vi "Initialize Session.vi"(8 "error in (no error)":errorcluster, 9 "Initialize_Info":T1, 10 "session reservation":refnum<class "Session Reservation.lvclass">, 11 "NI-DMM in":refnum<class "niDMM.lvclass">) -> (0 "error out":errorcluster, 3 "NI-DMM out":refnum<class "niDMM.lvclass">)   [LabVIEW 2021, in "niDMM.lvclass"]
uses:
  niDMM.lvclass
  TypeDefs/Initialize_Info.ctl
  <vilib>/Plug-In SDKs/Clients/Session Management V1/Session Reservation/Initialize and Close Session Behavior.ctl
  <vilib>/Plug-In SDKs/Clients/Session Management V1/Session Reservation/Session Reservation.lvclass
  niDMM.lvclass/niDMM.ctl
  <vilib>/Plug-In SDKs/Sessions/niDMM/Initialize Sessions - 1Sess.vi
  <vilib>/Plug-In SDKs/Sessions/niDMM/NI Session Management niDMM.lvlib
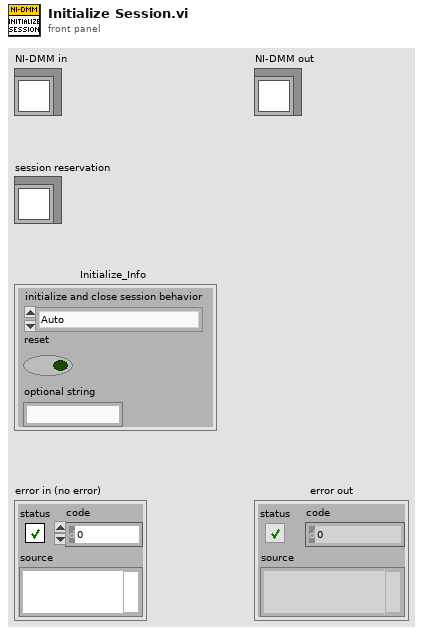
[diagram p1: front panel]
types:
  T1 = typedef "niDMM.lvclass/Initialize_Info.ctl" = cluster{"initialize and close session behavior":T2, "reset":bool, "optional string":string}
  T2 = typedef "NI Session Management V1 Client.lvlib/Session Reservation.lvclass/Initialize and Close Session Behavior.ctl" = enum16{"Auto", "Initialize and Close", "Attach and Detach", "Initialize and Detach", "Attach and Close"}
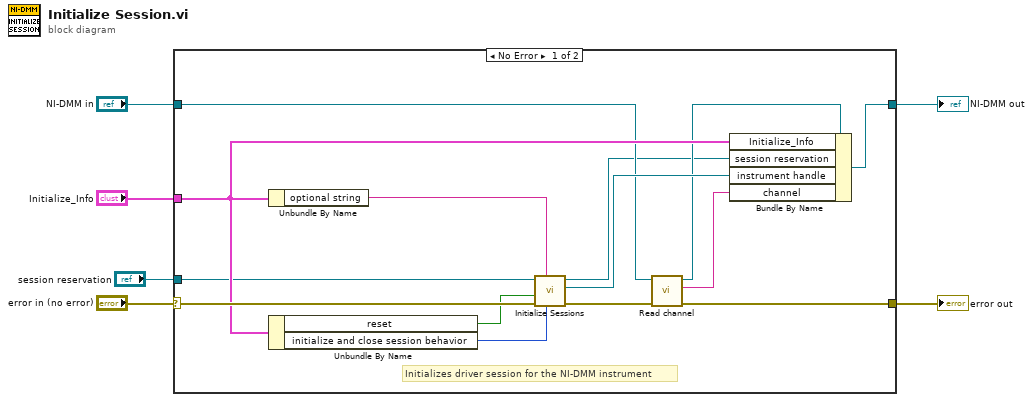
[diagram p0: block diagram]
diagram:
  n1 = case shown="No Error" "error in (no error)" {
    selector: "error in (no error)" -> [w19 w22]
    tunnel: "NI-DMM in" -> [w10 w21]
    tunnel: [w12 w22] -> w2
    tunnel: [w20 w21] -> w4
    tunnel: "Initialize_Info" -> [w14 _]
    tunnel: "session reservation" -> [w8 _]
    frame No Error {
      # "Initializes driver session for the NI-DMM instrument"
      n2 = Unbundle By Name(w14) -> ("optional string"=w15:string)
      n3 = Unbundle By Name(w14) -> ("reset"=w17:bool, "initialize and close session behavior"=w16:T2)
      n4 = call-poly <vilib>:"Initialize Sessions.vi"("initialize and close session behavior"=w16, "option string"=w15, "error in"=w19, "reset"=w17, "session reservation in"=w8) -> ("error out"=w13:errorcluster, "session"=w18:refnum<k15>, "session reservation out"=w7:refnum<class "Session Reservation.lvclass">)  [unwired: 3 in, 1 out]
      n5 = call-dynamic "Read channel.vi"("error in (no error)"=w13, "Abstract_Instrument in"=w10) -> ("error out"=w12:errorcluster, "channel"=w9:string, "Abstract_Instrument out"=w11:refnum<class "niDMM.lvclass">)  [unwired: 7 in]
      n6 = Bundle By Name(cluster=w11, "Initialize_Info"=w14, "session reservation"=w7, "instrument handle"=w18, "channel"=w9) -> (w20:refnum<class "niDMM.lvclass">)
    }
    frame Error {
    }
  }
  "NI-DMM out" <- w4
  "error out" <- w2
